vi "C1G2_Assemble Query Only.vi"(7 "Symbol Rate":dbl=10000000.0 format="%#_6p", 9 "Parameters Query":T2={"DR"=FALSE, "M"=1, "TRext (T=Pilot Tone)"=FALSE, "Sel"=1, "Session"=0, "Q"=0, "Target"=FALSE} {"Session" items=["S0", "S1", "S2", "S3"]; "Sel" items=["All", "All2", "~SL", "SL"]; "M" items=["M=1", "M=2", "M=4", "M=8"]}, 10 "Parameters Select":T3={"Target"=0, "Action"=0, "MemBank"=1, "truncate"=FALSE} {"MemBank" items=["00 RFU", "01 EPC", "10 TID", "11 User"]; "Action" items=["000", "001", "010", "011", "100", "101", "110", "111"]; "Target" items=["000 Inventoried (S0)", "001 Inventoried (S1)", "010 Inventoried (S2)", "011 Inventoried (S3)", "100 SL", "101 RFU", "110 RFU", "111 RFU"]}, 11 "Parameters Symbols":T1={"Tari"=8e-06, "PW"=0.5, "factor for \"1\" symbol"=0.5, "RTcal"=2.5, "TRcal"=3.0, "Delimiter"=1.25e-05} {"TRcal" min=1.1 max=3.0 step=0.1; "RTcal" min=2.5 max=3.0 step=0.1; "factor for \"1\" symbol" min=0.5 max=1.0 step=0.1; "PW" min=0.265 max=0.525 step=0.001; "Tari" format="%#_3p"}) -> (2 "Signal out":u8[](array[numeric]))   [LabVIEW 2015]
panel:
  in  "Select":bool
  out "CRC-16":u8[](array[numeric])=[1, 0, 1, 1, 0, 0, 0, 0, 0, 0, 0, 0, 0, 0, 0, 0] format="%0x"
  out "Query":i32
  out "CW":i32
  out "CRC-5":bool[](array[boolean])
  out "CRC-5":u8[](array[numeric])=[1, 0, 1, 1, 0] format="%0x"
  out "Symbols":i32=53374
  out "Digital Waveform":waveform(u8)(graph)={"t0"=timestamp(0 s since 1904-01-01), "dt"=1e-07, "Y"=array[53374 elements]}
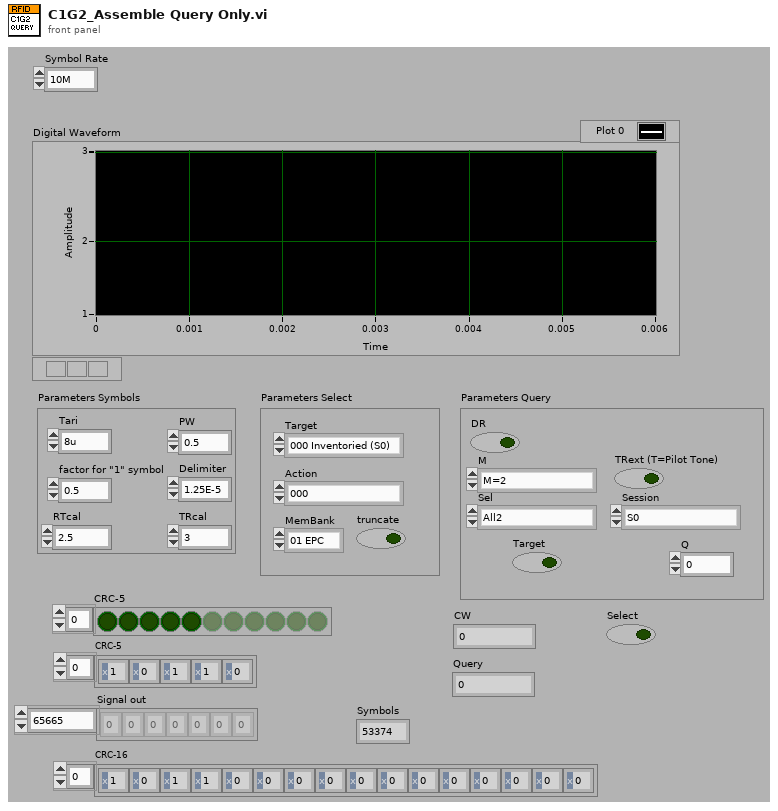
[diagram p1: front panel]
types:
  T1 = cluster{"Tari":dbl, "PW":dbl, "factor for \"1\" symbol":dbl, "RTcal":dbl, "TRcal":dbl, "Delimiter":dbl}
  T2 = cluster{"DR":bool, "M":u16, "TRext (T=Pilot Tone)":bool, "Sel":u16, "Session":u16, "Q":u8, "Target":bool}
  T3 = cluster{"Target":u16, "Action":u16, "MemBank":u16, "truncate":bool}
  T4 = typedef "C1G2_BasicsData.ctl" = cluster{"Symbol \"0\"":u8[], "Symbol \"1\"":u8[], "RT Preamble":u8[], "RT Frame Sync":u8[], "Sample Rate":dbl, "LOW-Pulse":u8[], "HIGH-Pulse":u8[], "RT cal":u8[]}
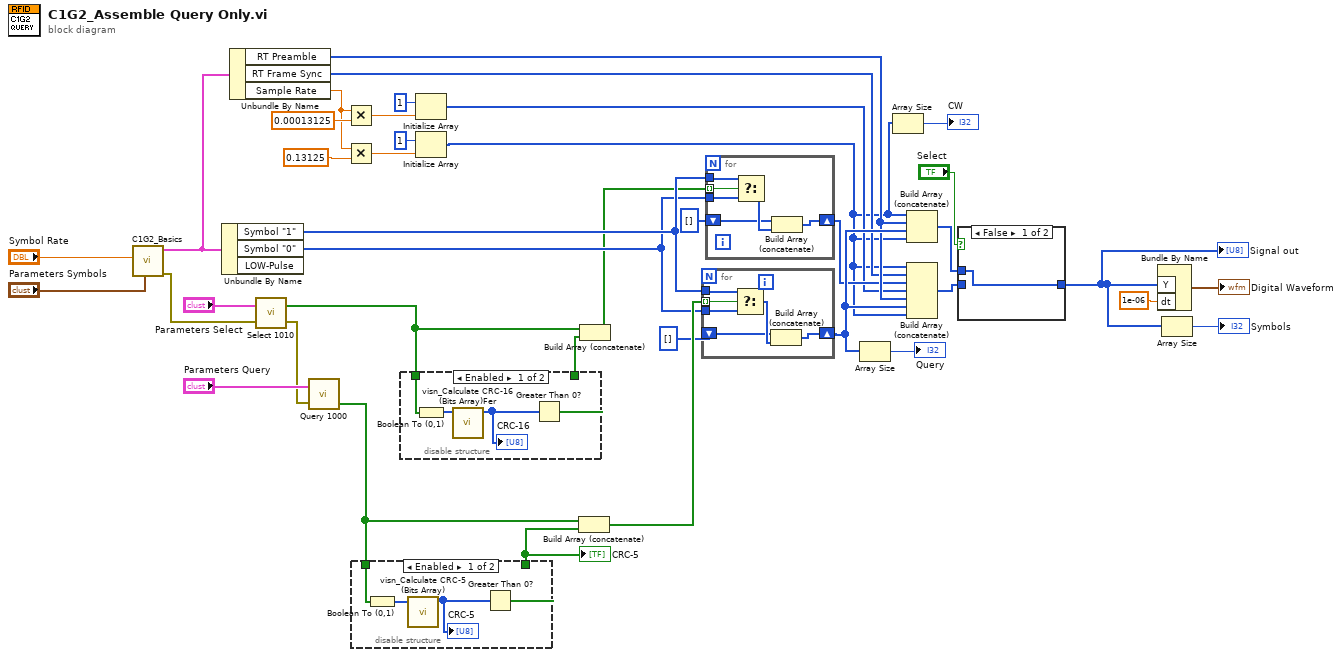
[diagram p0: block diagram]
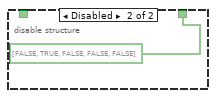
[diagram p3: hidden frame]
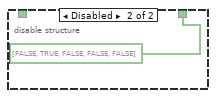
[diagram p4: hidden frame]
diagram:
  n1 = call "C1G2_Basics.vi"("Parameters Symbols"="Parameters Symbols", "Symbol Rate"="Symbol Rate") -> ("error out"=w23:errorcluster, "Basic Components"=w25:T4)  [unwired: 8 in]
  n2 = Unbundle By Name(w25) -> ("Symbol \"1\""=w20:u8[], "Symbol \"0\""=w19:u8[])  [unwired: 1 out]
  n3 = Unbundle By Name(w25) -> ("RT Preamble"=w10:u8[], "RT Frame Sync"=w4:u8[], "Sample Rate"=w12:dbl)
  n4 = call "Select 1010.vi"("error in (no error)"=w23, "Parameters Select"="Parameters Select") -> ("error out"=w22:errorcluster, "Array"=w13:bool[])
  n5 = call "Query 1000.vi"("error in (no error)"=w22, "Parameters Query"="Parameters Query") -> ("Array"=w15:bool[])  [unwired: 1 out]
  n6 = Multiply(x=w12, y=0.00013125 ("Pause length /s")) -> (x*y=w32:dbl)
  n7 = Multiply(x=w12, y=0.13125 ("Pause length /s")) -> (x*y=w28:dbl)
  n8 = disable-structure shown="Enabled" {
    disable-tunnel: w15 -> [w42 _]
    disable-tunnel: [w40 bool[] [FALSE, TRUE, FALSE, FALSE, FALSE]] -> w24
    frame Enabled {
      n9 = Boolean To (0,1)(Boolean=w42) -> (0, 1=w43:i16[])
      n10 = call "visn_Calculate CRC-5 (Bits Array).vi"("Bits Array"=w43) -> ("CRC-5"=w41:u8[])  [unwired: 10 in]
      "CRC-5" <- w41
      n11 = Greater Than 0?(x=w41) -> (x > 0?=w40:bool[])
    }
    frame Disabled {
    }
  }
  "CRC-5" <- w24
  n12 = disable-structure shown="Enabled" {
    disable-tunnel: w13 -> [w48 _]
    disable-tunnel: [w47 bool[] [FALSE, TRUE, FALSE, FALSE, FALSE]] -> w2
    frame Enabled {
      n13 = Boolean To (0,1)(Boolean=w48) -> (0, 1=w46:i16[])
      n14 = call "visn_Calculate CRC-16 (Bits Array)Fer.vi"("Bits Array"=w46) -> ("CRC-16"=w45:u8[])  [unwired: 10 in]
      "CRC-16" <- w45
      n15 = Greater Than 0?(x=w45) -> (x > 0?=w47:bool[])
    }
    frame Disabled {
    }
  }
  n16 = Initialize Array(u8 1 ("element"), w32) -> (w8:u8[])
  n17 = Initialize Array(u8 1 ("element"), w28) -> (w1:u8[])
  n18 = Build Array (concatenate)(w15, w24) -> (w21:bool[])
  n19 = Build Array (concatenate)(w13, w2) -> (w14:bool[])
  n20 = for {
    tunnel: w21 -> [w55] mode=indexing
    tunnel: w19 -> [w53]
    tunnel: w20 -> [w54]
    shift-right: [w52] -> w11
    shift-left: u8[] [] ("s? t:f") -> [w50]
    n21 = Select(t=w54, s=w55, f=w53) -> (s? t:f=w51:u8[])
    n22 = Build Array (concatenate)(w50, w51) -> (w52:u8[])
  }
  n23 = for {
    tunnel: w14 -> [w61] mode=indexing
    tunnel: w19 -> [w59]
    tunnel: w20 -> [w60]
    shift-right: [w58] -> w9
    shift-left: u8[] [] ("s? t:f") -> [w56]
    n24 = Select(t=w60, s=w61, f=w59) -> (s? t:f=w57:u8[])
    n25 = Build Array (concatenate)(w56, w57) -> (w58:u8[])
  }
  n26 = Array Size(array=w11) -> (size(s)=→"Query":i32)
  n27 = Array Size(array=w1) -> (size(s)=→"CW":i32)
  n28 = Build Array (concatenate)(w1, w10, w11, w1) -> (w7:u8[])
  n29 = Build Array (concatenate)(w1, w4, w9, w8, w10, w11, w1) -> (w6:u8[])
  n30 = case shown="False" "Select" {
    tunnel: w6 -> [_ w63]
    tunnel: [w62 w63] -> w3
    tunnel: w7 -> [w62 _]
    frame False {
    }
    frame True {
    }
  }
  "Signal out" <- w3
  n31 = Bundle By Name("Y"=w3, "dt"=1e-06) -> (→"Digital Waveform":waveform(u8))  [unwired: 1 in]
  n32 = Array Size(array=w3) -> (size(s)=→"Symbols":i32)
